vi "bg subtract array.vi"(3 "pix from edge":i32=2, 4 "Array":dbl[](array[numeric]), 5 "length 3":i32=200, 6 "length":i32=200) -> (0 "Average BG":dbl, 1 "Linearly interp BG":dbl[](array[numeric]), 2 "Output array BG subtracted":dbl[](graph))   [LabVIEW 2020]
uses:
  <vilib>/Analysis/1siggen.llb/Ramp Pattern by Samples.vi
  <vilib>/Analysis/NI_AALBase.lvlib
panel:
  in  "BG linear ramp":bool=TRUE
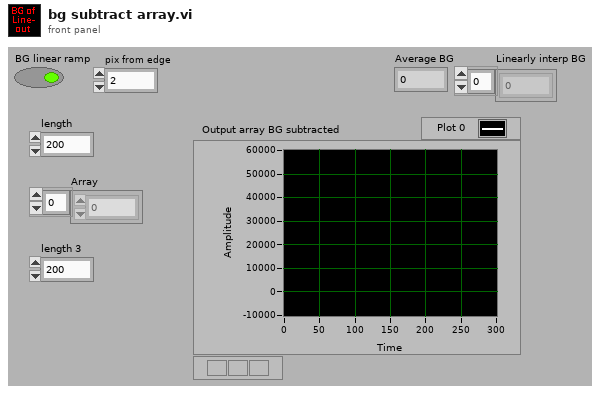
[diagram p1: front panel]
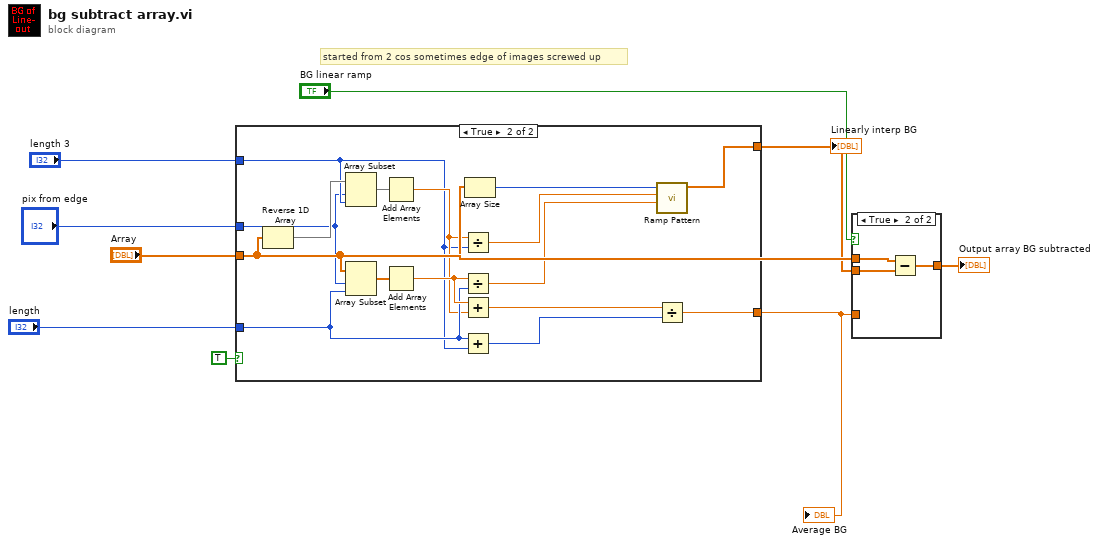
[diagram p0: block diagram]
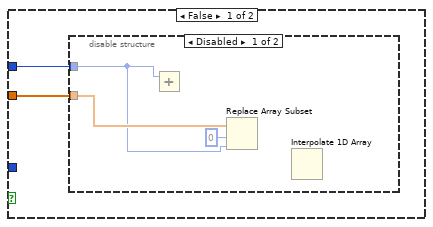
[diagram p2: hidden frame]
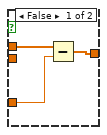
[diagram p4: hidden frame]
diagram:
  # "started from 2 cos sometimes edge of images screwed up"
  n1 = case shown="True" TRUE {
    tunnel: [_ w30] -> w8
    tunnel: "Array" -> [w11 w24]
    tunnel: "length" -> [_ w21]
    tunnel: "length 3" -> [_ w18]
    tunnel: [_ w16] -> w4
    tunnel: "pix from edge" -> [w10 w15]
    frame False {
      n2 = disable-structure shown="Disabled" {
        disable-tunnel: w11 -> [w14 _]
        disable-tunnel: w10 -> [w12 _]
        frame Disabled {
          n3 = Add(x=w12) -> ()  [unwired: 1 in, 1 out]
          n4 = Replace Array Subset(array=w14, new element=w12, index=0) -> ()  [unwired: 1 out]
          n5 = Interpolate 1D Array() -> ()  [unwired: 2 in, 1 out]
        }
        frame Enabled {
        }
      }
    }
    frame True {
      n6 = Reverse 1D Array(array=w24) -> (reversed array=w25:dbl[])
      n7 = Array Subset(array=w25, index=w15, length=w18) -> (w27:dbl[])
      n8 = Array Subset(array=w24, index=w15, length=w21) -> (w26:dbl[])
      n9 = Add Array Elements(numeric array=w27) -> (sum=w19:dbl)
      n10 = Add Array Elements(numeric array=w26) -> (sum=w22:dbl)
      n11 = Divide(x=w19, y=w18) -> (x/y=w17:dbl)
      n12 = Divide(x=w22, y=w21) -> (x/y=w20:dbl)
      n13 = Add(x=w22, y=w19) -> (x+y=w28:dbl)
      n14 = Add(x=w21, y=w18) -> (x+y=w29:i32)
      n15 = Array Size(array=w24) -> (size(s)=w23:i32)
      n16 = call-poly <vilib>:"Ramp Pattern.vi"("start"=w20, "end"=w17, "samples"=w23) -> ("Ramp Pattern"=w16:dbl[])  [unwired: 7 in, 1 out]
      n17 = Divide(x=w28, y=w29) -> (x/y=w30:dbl)
    }
  }
  "Average BG" <- w8
  "Linearly interp BG" <- w4
  n18 = case shown="True" "BG linear ramp" {
    tunnel: [w33 w34] -> w9
    tunnel: w8 -> [w32 _]
    tunnel: "Array" -> [w31 w36]
    tunnel: w4 -> [_ w35]
    frame False {
      n19 = Subtract(x=w31, y=w32) -> (x-y=w33:dbl[])
    }
    frame True {
      n20 = Subtract(x=w36, y=w35) -> (x-y=w34:dbl[])
    }
  }
  "Output array BG subtracted" <- w9
